vi "Error_Decompose Source String.vi"(11 "Error Source (String)":string) -> (2 "Call Chain":string, 3 "Description":string)   [LabVIEW 2019]
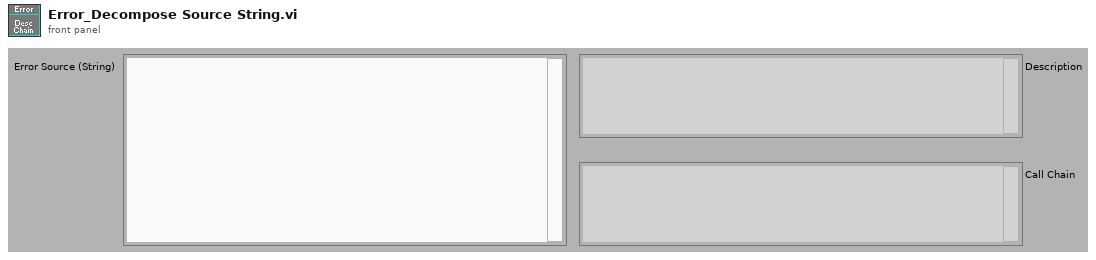
[diagram p1: front panel]
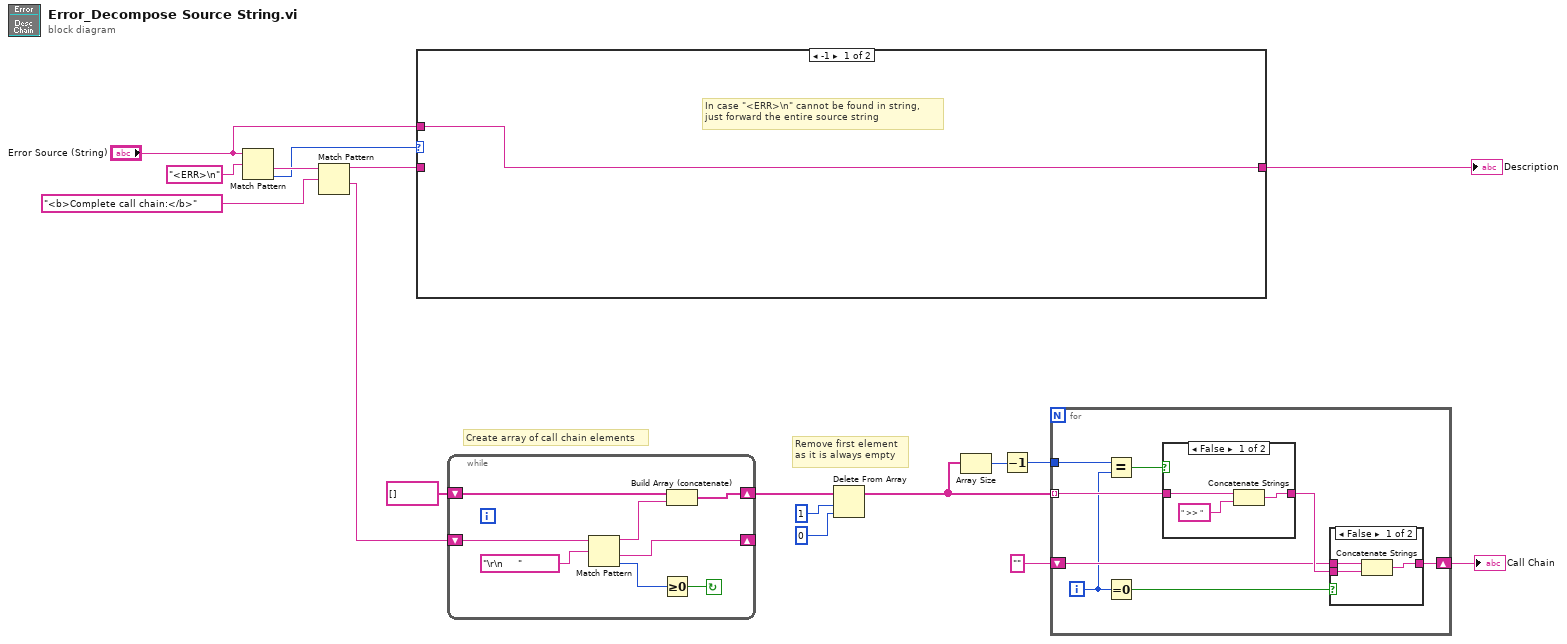
[diagram p0: block diagram]
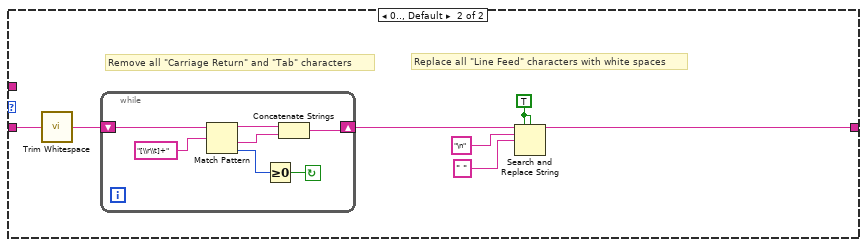
[diagram p2: hidden frame]
diagram:
  # "Remove first element\nas it is always empty"
  # "Create array of call chain elements"
  n1 = Match Pattern(string="Error Source (String)", regular expression="<ERR>\n") -> (after substring=w16:string, offset past match=w2:i32)  [unwired: 1 in, 2 out]
  n2 = Match Pattern(string=w16, regular expression="<b>Complete call chain:</b>") -> (before substring=w14:string, after substring=w13:string)  [unwired: 1 in, 2 out]
  n3 = case shown="-1" w2 {
    tunnel: w14 -> [_ w25]
    tunnel: [w18 w19] -> w3
    tunnel: "Error Source (String)" -> [w18 _]
    frame -1 {
      # "In case \"<ERR>\\n\" cannot be found in string,\njust forward the entire source string"
    }
    frame 0.., Default {
      w21 = TRUE ("replace all? (F)")
      # "Replace all \"Line Feed\" characters with white spaces"
      # "Remove all \"Carriage Return\" and \"Tab\" characters"
      n4 = call <vilib>:"Trim Whitespace.vi"("string"=w25) -> ("trimmed string"=w20:string)  [unwired: 1 in]
      n5 = while {
        shift-right: [w27] -> w24
        shift-left: w20 -> [w32]
        stop <- w30 continue-if-true
        n6 = Match Pattern(string=w32, regular expression="[\\r\\t]+") -> (before substring=w29:string, after substring=w28:string, offset past match=w31:i32)  [unwired: 2 out]
        n7 = Greater Or Equal To 0?(x=w31) -> (x >= 0?=w30:bool)
        n8 = Concatenate Strings(w29, w28) -> (w27:string)
      }
      n9 = Search and Replace String(replace all?=w21, case sensitive?=w21, input string=w24, search string="\n", replace string=" " ("replace string (\"\")")) -> (result string=w19:string)  [unwired: 3 in, 3 out]
    }
  }
  "Description" <- w3
  n10 = while {
    shift-right: [w36] -> _
    shift-left: w13 -> [w40]
    shift-right: [w34] -> w9
    shift-left: string[] [] -> [w33]
    stop <- w37 continue-if-true
    n11 = Match Pattern(string=w40, regular expression="\r\n     ") -> (before substring=w35:string, after substring=w36:string, offset past match=w39:i32)  [unwired: 2 out]
    n12 = Greater Or Equal To 0?(x=w39) -> (x >= 0?=w37:bool)
    n13 = Build Array (concatenate)(w33, w35) -> (w34:string[])
  }
  n14 = Delete From Array(array=w9, length=1, index=0) -> (array with subset deleted=w6:string[])  [unwired: 1 out]
  n15 = Array Size(array=w6) -> (size(s)=w5:i32)
  n16 = Decrement(x=w5) -> (x-1=w4:i32)
  n17 = for {
    tunnel: w6 -> [w48] mode=indexing
    shift-right: [w45] -> w10
    shift-left: "" -> [w46]
    tunnel: w4 -> [w43]
    i -> [w42]
    n18 = Equal?(x=w43, y=w42) -> (x = y?=w41:bool)
    n19 = Equal To 0?(x=w42) -> (x = 0?=w44:bool)
    n20 = case shown="False" w41 {
      tunnel: w48 -> [w55 w56]
      tunnel: [w53 w56] -> w47
      frame False {
        n21 = Concatenate Strings(w55, " >> " ("string")) -> (w53:string)
      }
      frame True {
      }
    }
    n22 = case shown="False" w44 {
      tunnel: w47 -> [w51 _]
      tunnel: w46 -> [w50 w52]
      tunnel: [w49 w52] -> w45
      frame False {
        n23 = Concatenate Strings(w50, w51) -> (w49:string)
      }
      frame True {
      }
    }
  }
  "Call Chain" <- w10
